vi "例程48-状态机.vi"() -> ()   [LabVIEW 2016]
panel:
  out "枚举":enum16{"INIT", "DAQ", "STOP"}(ring)
  in  "停止":bool
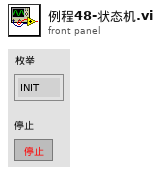
[diagram p1: front panel]
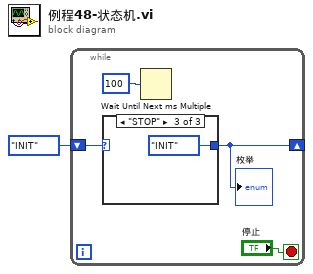
[diagram p0: block diagram]
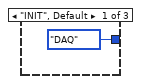
[diagram p2: hidden frame]
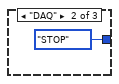
[diagram p3: hidden frame]
diagram:
  n1 = while {
    shift-right: [w4] -> _
    shift-left: enum16{"INIT", "DAQ", "STOP"}."INIT" ("枚举") -> [w5]
    stop <- "停止" stop-if-true
    n2 = case shown="\"STOP\"" w5 {
      tunnel: [enum16{"INIT", "DAQ", "STOP"}."DAQ" ("枚举") enum16{"INIT", "DAQ", "STOP"}."STOP" ("枚举") enum16{"INIT", "DAQ", "STOP"}."INIT" ("枚举")] -> w4
      frame "INIT", Default {
      }
      frame "DAQ" {
      }
      frame "STOP" {
      }
    }
    "枚举" <- w4
    n3 = Wait Until Next ms Multiple(millisecond multiple=u32 100 ("毫秒倍数")) -> ()  [unwired: 1 out]
  }
